vi "TBM root configuration version.vi"() -> (3 "version":string="1.0.0.0")   [LabVIEW 2013, in "TBM configuration.lvclass"]
uses:
  TBM configuration.lvclass
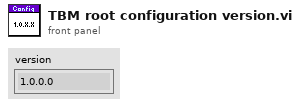
[diagram p1: front panel]
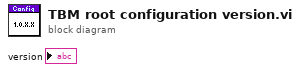
[diagram p0: block diagram]
diagram:
